vi "CIE Lab Color Distance.vi"() -> ()   [LabVIEW 2014]
doc: "This example shows how to use color space conversions to measure the distance, or difference, between two colors."
uses:
  <vilib>/vision/NI_Vision_Development_Module.lvlib
panel:
  out "Color Distance (CIE L*a*b*)":dbl format="%.2f"
  in  "Stop":bool
  out "2D Color Triangle":T1(plugin-control)
  out "Color Image":T1(plugin-control)
  # "Overview: Demonstrates how to use the IMAQ RGBToColor function to convert RGB values to CIE L*a*b* and XYZ points so the Color Distance can be calculated and the location on the 2D Color Triangle can be shown.\nRequirements: Vision Development Software.\nInstructions:\n1. Run the VI.\n2. Click on the Color Image to update the points used to calculate the color distance. The 2D Color Triangle is used to show where those colors are located in the XYZ space."
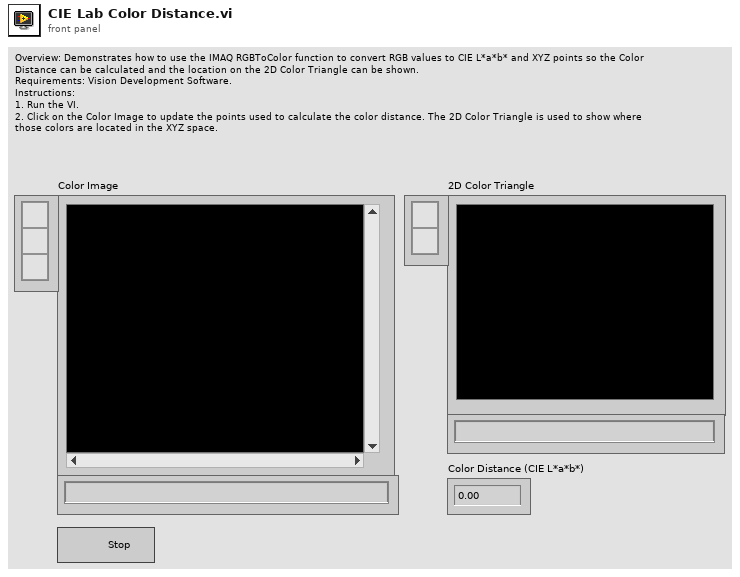
[diagram p1: front panel]
types:
  T1 = typedef "IMAQ Image.ctl" = refnum<image>
  T2 = typedef "Image Type" = u32
  T3 = cluster{"Coordinates[0]":i32, "Coordinates[1]":i32}
  T4 = cluster{"Coordinates[0]":i32, "Coordinates[1]":i32}[]
  T5 = cluster{"Red (or Hue) value":u8, "Green (or Sat) value":u8, "Blue (or Light or Val) value":u8}
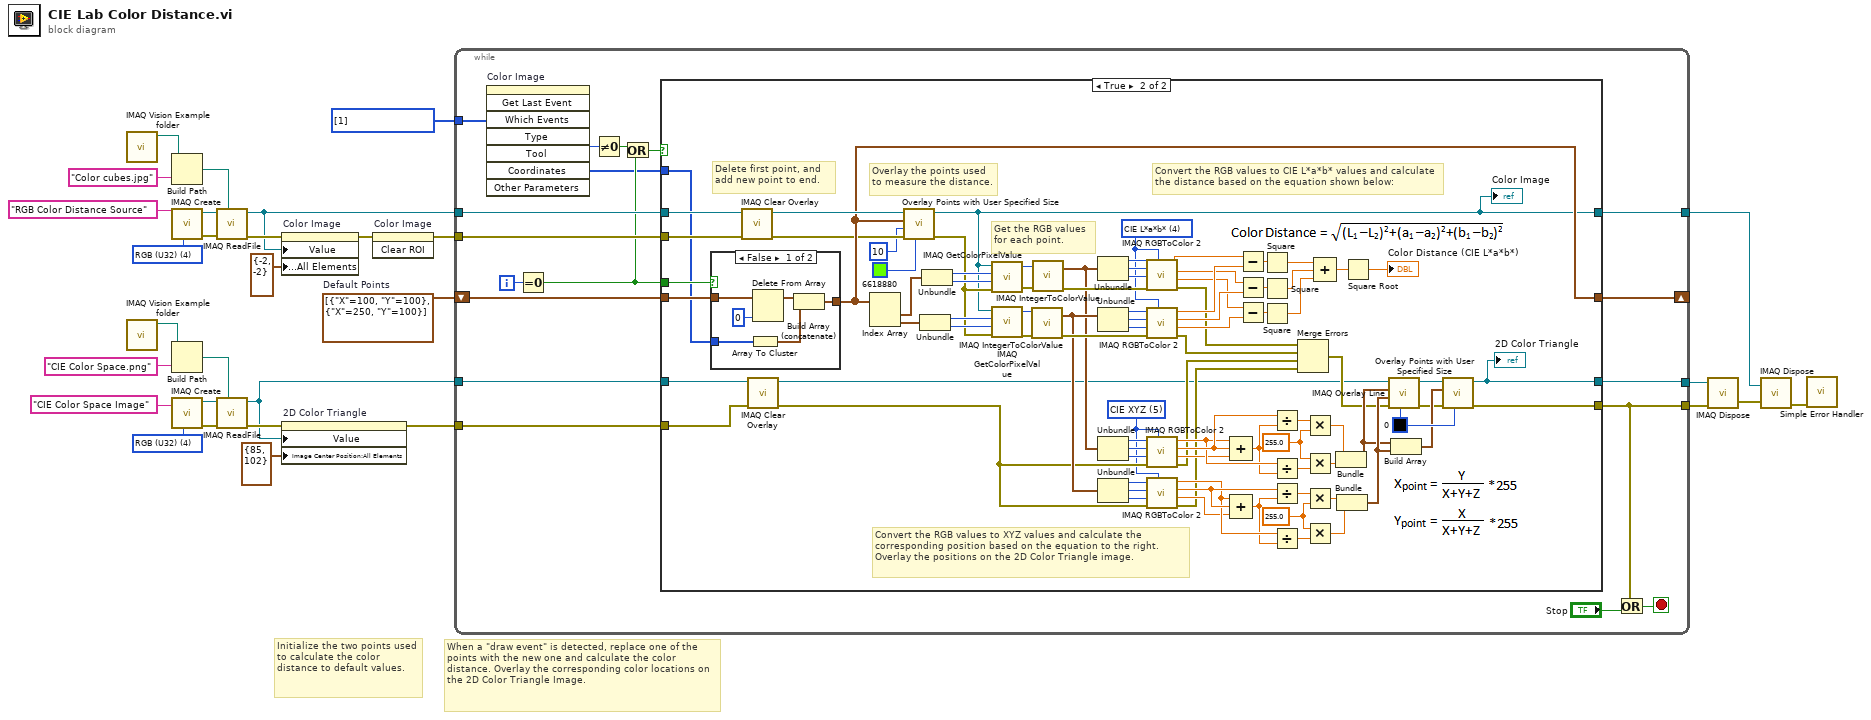
[diagram p0: block diagram]
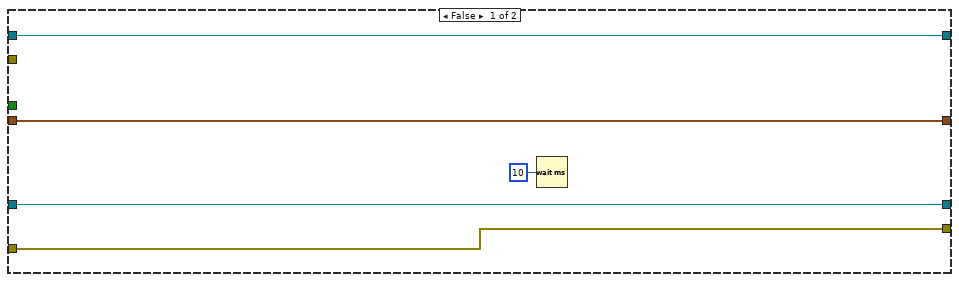
[diagram p2: hidden frame]
diagram:
  w4 = T2 4 items=["Grayscale (U8)", "Grayscale (I16)", "Grayscale (SGL)", "Complex (CSG)", "RGB (U32)", "HSL (U32)", "RGB (U64)", "Grayscale (U16)"] ("Image Type")
  w5 = T2 4 items=["Grayscale (U8)", "Grayscale (I16)", "Grayscale (SGL)", "Complex (CSG)", "RGB (U32)", "HSL (U32)", "RGB (U64)", "Grayscale (U16)"] ("Image Type")
  w10 = i32[] [1] items=["No Event"=0, "Click Event"=1, "Draw Event"=2, "Size Event"=4, "Scroll Event"=5, "Double Click Event"=8] ("Which Events")
  w12 = cluster{"X":i32, "Y":i32}[] [{"X"=100, "Y"=100}, {"X"=250, "Y"=100}]  # Default Points
  # "Initialize the two points used to calculate the color distance to default values."
  # "When a \"draw event\" is detected, replace one of the points with the new one and calculate the color distance. Overlay the corresponding color locations on the 2D Color Triangle Image."
  n1 = call "IMAQ Vision Example folder.vi"() -> ("Example Image Path"=w27:path)  [unwired: 11 in]
  n2 = call "IMAQ Vision Example folder.vi"() -> ("Example Image Path"=w21:path)  [unwired: 11 in]
  n3 = Build Path(base path=w27, name or relative path="Color cubes.jpg") -> (appended path=w25:path)
  n4 = call "IMAQ Create"("Image Name"="RGB Color Distance Source", "Image Type"=w4) -> ("New Image"=w29:T1, "error out"=w28:errorcluster)  [unwired: 3 in]
  n5 = Build Path(base path=w21, name or relative path="CIE Color Space.png") -> (appended path=w19:path)
  n6 = call "IMAQ Create"("Image Name"="CIE Color Space Image", "Image Type"=w5) -> ("New Image"=w2:T1, "error out"=w22:errorcluster)  [unwired: 3 in]
  n7 = call "IMAQ ReadFile"("File Path"=w25, "error in (no error)"=w28, "Image"=w29) -> ("error out"=w15:errorcluster, "Image Out"=w11:T1)  [unwired: 4 in, 3 out]
  n8 = call "IMAQ ReadFile"("File Path"=w19, "error in (no error)"=w22, "Image"=w2) -> ("error out"=w13:errorcluster, "Image Out"=w1:T1)  [unwired: 4 in, 3 out]
  n9 = property on="Color Image" class="ImageControl"(error in=w15, "Value"=w11, "ZoomInteger:All Elements"=cluster{"X":i32, "Y":i32} {"X"=-2, "Y"=-2} ("Zoom:All Elements")) -> (error out=w17:errorcluster)  [unwired: 1 in, 1 out]
  n10 = property on="2D Color Triangle" class="ImageControl"(error in=w13, "Value"=w1, "Image Center Position:All Elements"=cluster{"X":u32, "Y":u32} {"X"=85, "Y"=102}) -> (error out=w16:errorcluster)  [unwired: 1 in, 1 out]
  n11 = invoke on="Color Image" class="ImageControl" method="Clear ROI"(error in=w17) -> (error out=w14:errorcluster)  [unwired: 2 in, 2 out]
  n12 = while {
    tunnel: w11 -> [w45]
    tunnel: w1 -> [w34]
    tunnel: w16 -> [w43]
    tunnel: w14 -> [w44]
    shift-right: [w46] -> _
    shift-left: w12 -> [w48]
    tunnel: w10 -> [w47]
    tunnel: [w32] -> w9
    tunnel: [w33] -> w8
    tunnel: [w41] -> w6
    i -> [w38]
    stop <- w40 stop-if-true
    n13 = invoke on="Color Image" class="ImageControl" method="Get Last Event"("Which Events"=w47) -> ("Tool"=w37:i32, "Coordinates"=w31:i32[])  [unwired: 7 in, 6 out]
    n14 = Equal To 0?(x=w38) -> (x = 0?=w35:bool)
    n15 = Not Equal To 0?(x=w37) -> (x != 0?=w36:bool)
    n16 = Or(x=w36, y=w35) -> (x .or. y?=w39:bool)
    n17 = case shown="True" w39 {
      tunnel: w45 -> [w50 w95]
      tunnel: w34 -> [w49 w96]
      tunnel: w48 -> [w52 w87]
      tunnel: [w52 w86] -> w46
      tunnel: w31 -> [_ w54]
      tunnel: w44 -> [_ w83]
      tunnel: w43 -> [w51 w82]
      tunnel: [w51 w66] -> w41
      tunnel: w35 -> [_ w62]
      tunnel: [w50 w60] -> w33
      tunnel: [w49 w59] -> w32
      frame False {
        n18 = Wait (ms)(milliseconds to wait=u32 10) -> ()  [unwired: 1 out]
      }
      frame True {
        w126 = u32 0 ("Color")
        w106 = 255.0 ("y")
        w57 = u16 5 items=["RGB", "HSL", "HSV", "HSI", "CIE L*a*b*", "CIE XYZ"] ("Color Mode")
        w101 = 255.0 ("y")
        w58 = u16 4 items=["RGB", "HSL", "HSV", "HSI", "CIE L*a*b*", "CIE XYZ"] ("Color Mode")
        # "Delete first point, and add new point to end."
        # "Convert the RGB values to XYZ values and calculate the corresponding position based on the equation to the right. Overlay the positions on the 2D Color Triangle image."
        # "Convert the RGB values to CIE L*a*b* values and calculate the distance based on the equation shown below:"
        # "Get the RGB values for each point."
        # "Overlay the points used to measure the distance."
        n19 = case shown="False" w62 {
          tunnel: w87 -> [w148 w149]
          tunnel: [w145 w149] -> w86
          tunnel: w54 -> [w144 _]
          frame False {
            n20 = Array To Cluster(array=w144) -> (cluster=w143:T3)
            n21 = Delete From Array(array=w148, index=0) -> (array with subset deleted=w146:cluster{"X":i32, "Y":i32}[])  [unwired: 1 in, 1 out]
            n22 = Build Array (concatenate)(w146, w143) -> (w145:T4)
          }
          frame True {
            # "Use default point values"
          }
        }
        n23 = call "IMAQ Clear Overlay"("error in (no error)"=w83, "Image"=w95) -> ("error out"=w81:errorcluster, "Image Out"=w88:T1)  [unwired: 8 in]
        n24 = call "IMAQ Clear Overlay"("error in (no error)"=w82, "Image"=w96) -> ("error out"=w79:errorcluster, "Image Out"=w65:T1)  [unwired: 8 in]
        n25 = Index Array(array=w86) -> (element #1=w94:cluster{"X":i32, "Y":i32}, element #2=w91:cluster{"X":i32, "Y":i32})  [unwired: 2 in]
        n26 = call "Overlay Points with User Specified Size.vi"("Color"=u32 6618880, "error in"=w81, "Point Diameter (5)"=u32 10 ("Point Size (5)"), "Points"=w86, "Image In"=w88) -> ("error out"=w80:errorcluster, "Image Out"=w60:T1)  [unwired: 5 in]
        "Color Image" <- w60
        n27 = Unbundle(w91) -> ("X"=w90:i32, "Y"=w89:i32)
        n28 = Unbundle(w94) -> ("X"=w93:i32, "Y"=w92:i32)
        n29 = call "IMAQ GetColorPixelValue"("error in (no error)"=w80, "Y Coordinate"=w92, "X Coordinate"=w93, "Image"=w60) -> ("error out"=w84:errorcluster, "Pixel Value (U32)"=w139:u32)  [unwired: 1 out]
        n30 = call "IMAQ GetColorPixelValue"("error in (no error)"=w80, "Y Coordinate"=w89, "X Coordinate"=w90, "Image"=w60) -> ("error out"=w55:errorcluster, "Pixel Value (U32)"=w140:u32)  [unwired: 1 out]
        n31 = call "IMAQ IntegerToColorValue"("error in (no error)"=w55, "U32 value"=w140) -> ("error out"=w141:errorcluster, "Color Value"=w98:T5)  [unwired: 3 in, 2 out]
        n32 = call "IMAQ IntegerToColorValue"("error in (no error)"=w84, "U32 value"=w139) -> ("error out"=w142:errorcluster, "Color Value"=w97:T5)  [unwired: 3 in, 2 out]
        n33 = Unbundle(w97) -> ("Red (or Hue) value"=w127:u8, "Green (or Sat) value"=w130:u8, "Blue (or Light or Val) value"=w132:u8)
        n34 = Unbundle(w98) -> ("Red (or Hue) value"=w129:u8, "Green (or Sat) value"=w128:u8, "Blue (or Light or Val) value"=w131:u8)
        n35 = Unbundle(w97) -> ("Red (or Hue) value"=w114:u8, "Green (or Sat) value"=w115:u8, "Blue (or Light or Val) value"=w116:u8)
        n36 = Unbundle(w98) -> ("Red (or Hue) value"=w117:u8, "Green (or Sat) value"=w118:u8, "Blue (or Light or Val) value"=w119:u8)
        n37 = call "IMAQ RGBToColor 2"("Color Mode"=w58, "error in (no error)"=w142, "Blue value"=w132, "Green value"=w130, "Red value"=w127) -> ("error out"=w78:errorcluster, "Blue or Luma or Val or Inten or Z or b*value"=w133:dbl, "Green or Sat or Y or a* value"=w56:dbl, "Red or Hue or X or L* value"=w137:dbl)  [unwired: 3 in]
        n38 = call "IMAQ RGBToColor 2"("Color Mode"=w58, "error in (no error)"=w141, "Blue value"=w131, "Green value"=w128, "Red value"=w129) -> ("error out"=w77:errorcluster, "Blue or Luma or Val or Inten or Z or b*value"=w134:dbl, "Green or Sat or Y or a* value"=w135:dbl, "Red or Hue or X or L* value"=w136:dbl)  [unwired: 3 in]
        n39 = call "IMAQ RGBToColor 2"("Color Mode"=w57, "error in (no error)"=w79, "Blue value"=w116, "Green value"=w115, "Red value"=w114) -> ("error out"=w70:errorcluster, "Blue or Luma or Val or Inten or Z or b*value"=w103:dbl, "Green or Sat or Y or a* value"=w120:dbl, "Red or Hue or X or L* value"=w111:dbl)  [unwired: 3 in]
        n40 = call "IMAQ RGBToColor 2"("Color Mode"=w57, "error in (no error)"=w79, "Blue value"=w119, "Green value"=w118, "Red value"=w117) -> ("error out"=w69:errorcluster, "Blue or Luma or Val or Inten or Z or b*value"=w108:dbl, "Green or Sat or Y or a* value"=w113:dbl, "Red or Hue or X or L* value"=w112:dbl)  [unwired: 3 in]
        n41 = Compound Arithmetic op=ADD(w111, w120, w103) -> (w99:dbl)
        n42 = Compound Arithmetic op=ADD(w112, w113, w108) -> (w104:dbl)
        n43 = Subtract(x=w137, y=w136) -> (x-y=w76:dbl)
        n44 = Subtract(x=w56, y=w135) -> (x-y=w74:dbl)
        n45 = Subtract(x=w133, y=w134) -> (x-y=w73:dbl)
        n46 = Square(x=w76) -> (x^2=w75:dbl)
        n47 = Square(x=w74) -> (x^2=w71:dbl)
        n48 = Square(x=w73) -> (x^2=w72:dbl)
        n49 = Divide(x=w120, y=w99) -> (x/y=w100:dbl)
        n50 = Divide(x=w111, y=w99) -> (x/y=w102:dbl)
        n51 = Divide(x=w113, y=w104) -> (x/y=w105:dbl)
        n52 = Divide(x=w112, y=w104) -> (x/y=w107:dbl)
        n53 = Merge Errors(w78, w77, w70, w69) -> (w68:errorcluster)
        n54 = Multiply(x=w100, y=w101) -> (x*y=w109:dbl)
        n55 = Multiply(x=w101, y=w102) -> (x*y=w110:dbl)
        n56 = Multiply(x=w105, y=w106) -> (x*y=w121:dbl)
        n57 = Multiply(x=w106, y=w107) -> (x*y=w122:dbl)
        n58 = Compound Arithmetic op=ADD(w75, w71, w72) -> (w138:dbl)
        n59 = Bundle(w109, w110) -> (w123:cluster{dbl, dbl})  [unwired: 1 in]
        n60 = Bundle(w121, w122) -> (w125:cluster{dbl, dbl})  [unwired: 1 in]
        n61 = Square Root(x=w138) -> (sqrt(x)=→"Color Distance (CIE L*a*b*)":dbl)
        n62 = call "IMAQ Overlay Line"("Color"=w126, "error in (no error)"=w68, "End Point"=w125, "Start Point"=w123, "Image"=w65) -> ("error out"=w67:errorcluster, "Image Out"=w64:T1)  [unwired: 5 in]
        n63 = Build Array(w123, w125) -> (w124:cluster{dbl, dbl}[])
        n64 = call "Overlay Points with User Specified Size.vi"("Color"=w126, "error in"=w67, "Points"=w124, "Image In"=w64) -> ("error out"=w66:errorcluster, "Image Out"=w59:T1)  [unwired: 6 in]
        "2D Color Triangle" <- w59
      }
    }
    n65 = Or(x=w41, y="Stop") -> (x .or. y?=w40:bool)
  }
  n66 = call "IMAQ Dispose"("Image"=w9, "error in (no error)"=w6) -> ("error out"=w7:errorcluster)  [unwired: 4 in]
  n67 = call "IMAQ Dispose"("Image"=w8, "error in (no error)"=w7) -> ("error out"=w3:errorcluster)  [unwired: 4 in]
  n68 = call <vilib>:"Simple Error Handler.vi"("error in (no error)"=w3) -> ()  [unwired: 4 in, 5 out]
